vi "Publish Message.vi"(8 "error in (no error)":errorcluster, 9 "Message Priority (Normal)":T1=enum."Normal", 10 "Message to Publish":refnum<class "Message.lvclass">, 11 "Actor in":refnum<class "Actor.lvclass">) -> (0 "error out":errorcluster, 1 "Dropped?":bool, 3 "Actor out":refnum<class "Actor.lvclass">)   [LabVIEW 2020, in "Publisher.lvlib" / "Publish Msg.lvclass"]
doc: "This VI sends the message to an actor."
uses:
  Publish Msg.lvclass
  PPL/HDH.Actor Framework.Core.Actor.lvlibp/1abvi3w/vi.lib/ActorFramework/Actor/Actor.lvclass
  PPL/HDH.Actor Framework.Core.Actor.lvlibp/1abvi3w/vi.lib/ActorFramework/Message Enqueuer/Message Priority.ctl
  PPL/HDH.Actor Framework.Core.Actor.lvlibp/1abvi3w/vi.lib/ActorFramework/Message/Message.lvclass
  C:/Current projects/WS/Framework/Framework/Actors/Publisher/Publisher Messages/Publisher Msg/Publisher Msg.lvclass
  Publish Msg.lvclass/Publish Msg.ctl
  Publisher Msg/Publisher Msg.lvclass
  PPL/HDH.Actor Framework.Core.Actor.lvlibp/1abvi3w/vi.lib/ActorFramework/Message Enqueuer/Message Enqueuer.lvclass
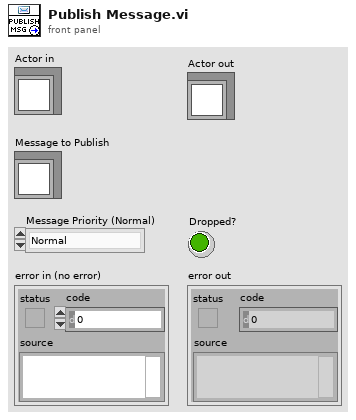
[diagram p1: front panel]
types:
  T1 = typedef "HDH.Actor Framework.Core.Actor.lvlibp/Message Enqueuer.lvclass/Message Priority.ctl" = enum16{"Low", "Normal", "High"}
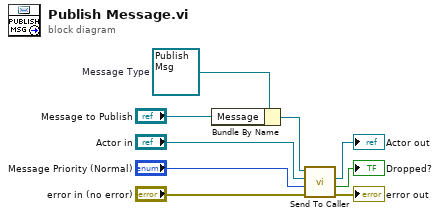
[diagram p0: block diagram]
diagram:
  w9 = refnum<class "Publish Msg.lvclass"> refnum  # Message Type
  n1 = Bundle By Name(cluster=w9, "Message"="Message to Publish") -> (w3:refnum<class "Publish Msg.lvclass">)
  n2 = call "Send To Caller.vi"("error in (no error)"="error in (no error)", "Message Priority (Normal)"="Message Priority (Normal)", "Actor in"="Actor in", "Publisher Msg in"=w3) -> ("error out"=→"error out":errorcluster, "Msg Dropped?"=→"Dropped?":bool, "Actor out"=→"Actor out":refnum<class "Actor.lvclass">)  [unwired: 5 in]
